vi "garphic 2.vi"() -> ()   [LabVIEW 2019]
panel:
  in  "Tab Control":T1(tab)
  in  "Slide":dbl(slide) scale=0.0..10.0
  out "Thermometer":dbl(slide) scale=0.0..100.0
  in  "Tab Control 2":enum32{"Page 1", "Page 2"}(tab)
  out "Meter":cluster{dbl, dbl}(knob) scale=0.0..10.0
  out "Gauge":dbl(knob) scale=0.0..10.0
  out "Waveform Chart":dbl(graph)
  in  "Boolean 13":bool
  out "Boolean 9":bool
  in  "Cancel Button":bool
  in  "OK Button 2":bool
  in  "OK Button":bool
  in  "Boolean 8":bool
  out "Boolean 7":bool
  out "Boolean 6":bool
  in  "Boolean 5":bool
  out "Boolean 4":bool
  out "Boolean 3":bool
  out "Numeric":dbl
  out "Boolean 12":bool
  out "Boolean 2":bool
  out "Boolean":bool
  out "Boolean 11":bool
  out "Boolean 10":bool
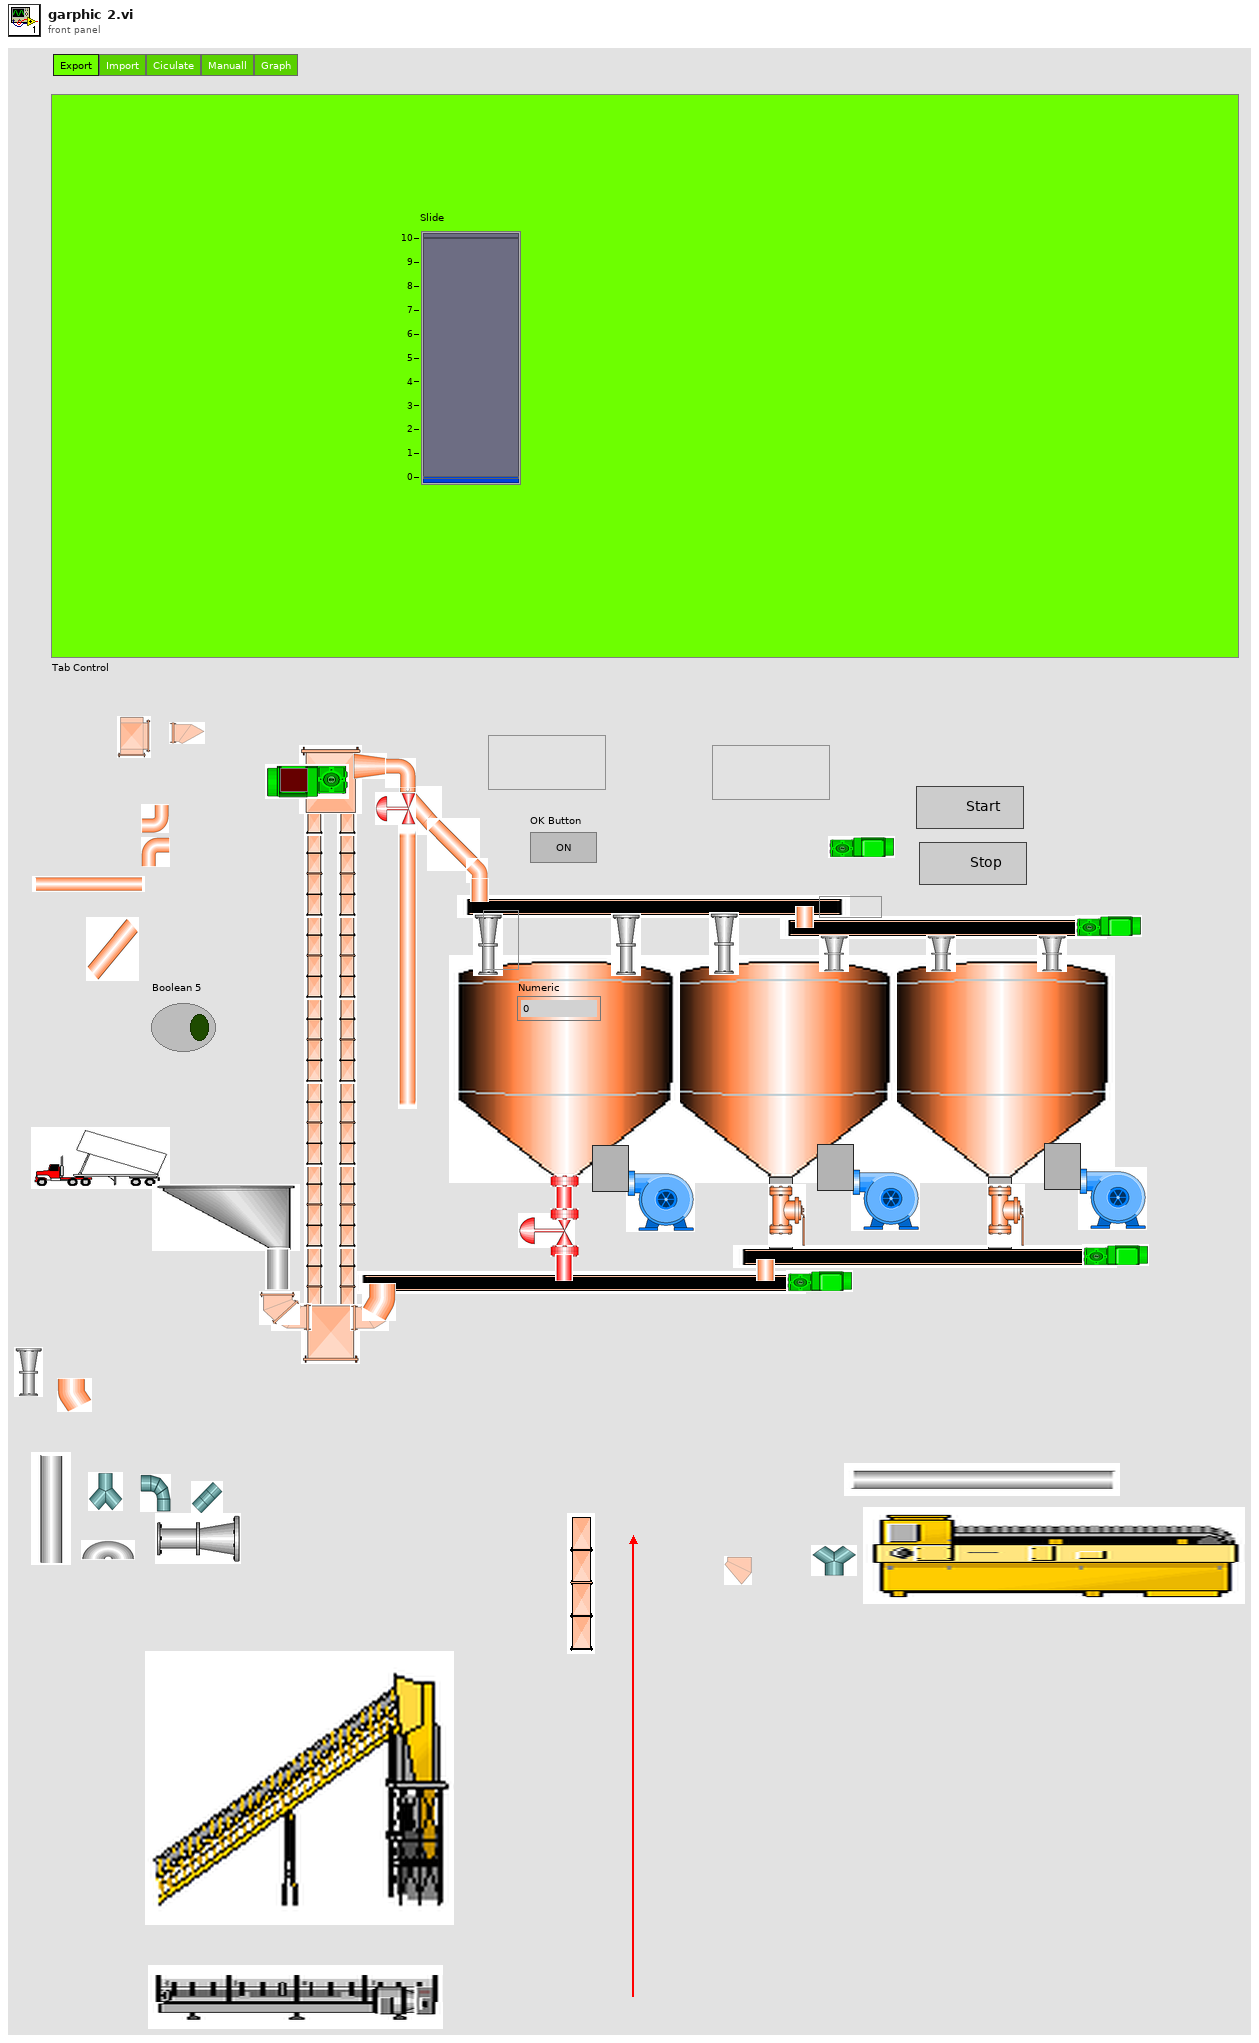
[diagram p1: front panel]
types:
  T1 = enum32{"Export", "Import", "Ciculate", "Manuall", "Graph"}
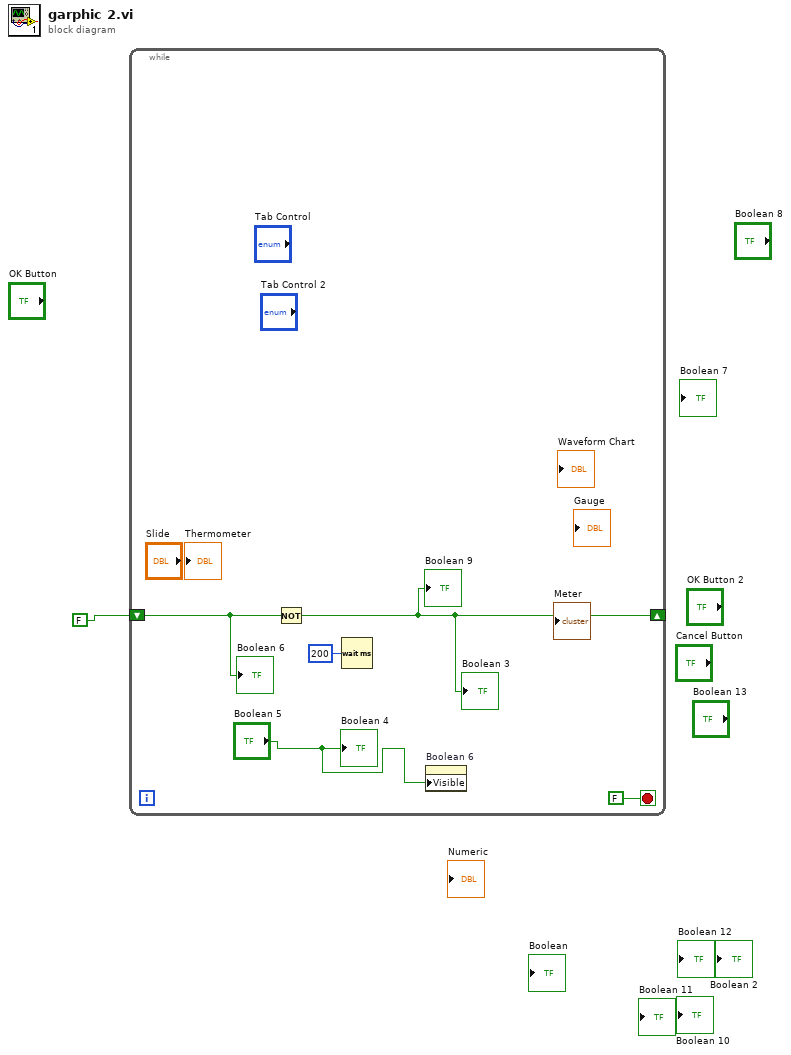
[diagram p0: block diagram]
diagram:
  n1 = while {
    shift-right: [w2] -> _
    shift-left: FALSE -> [w3]
    stop <- FALSE stop-if-true
    n2 = Not(x=w3) -> (.not. x?=w2:bool)
    "Boolean 3" <- w2
    "Boolean 9" <- w2
    n3 = Wait (ms)(milliseconds to wait=u32 200) -> ()  [unwired: 1 out]
    n4 = property on="Boolean 6" class="Bool (strict)"("Visible"="Boolean 5") -> ()  [unwired: 2 in, 2 out]
    "Boolean 4" <- "Boolean 5"
    "Boolean 6" <- w3
  }
